vi "USB_test.vi"() -> ()   [LabVIEW 2024]
uses:
  <vilib>/Instr/_visa.llb/VISA Configure Serial Port (Instr).vi
panel:
  out "return count 2":u32
  in  "timeout (10sec)":u32=10000
  out "return count":u32
  out "error out":errorcluster
  out "read buffer":string
  in  "error in (no error)":errorcluster
  in  "VISA resource name":refnum<visa-resource-name>
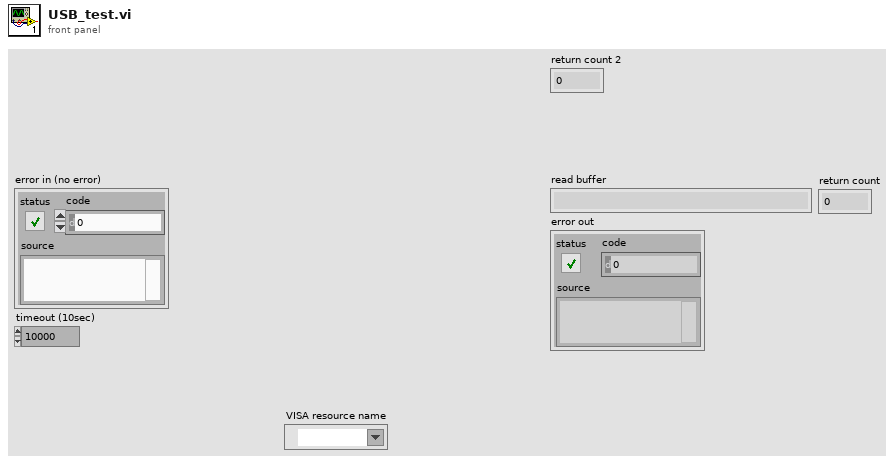
[diagram p1: front panel]
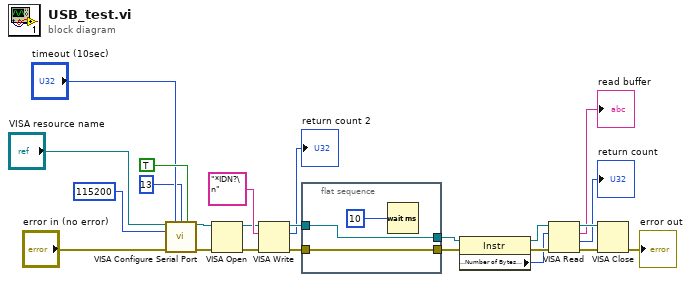
[diagram p0: block diagram]
diagram:
  n1 = call-poly "VISA Configure Serial Port"("VISA resource name"="VISA resource name", "timeout (10sec)"="timeout (10sec)", "termination char\n(0xA = '\\n' = LF)"=u8 13 ("termination char\n(0xA = '\\n' = LF)"), "Enable Termination\nChar (T)"=TRUE ("Enable Termination\nChar (T)"), "baud rate (9600)"=u32 115200, "error in (no error)"="error in (no error)") -> ("VISA resource name out"=w5:refnum<visa-resource-name>, "error out"=w6:errorcluster)  [unwired: 8 in]
  n2 = VISA Open(error in (no error)=w6, VISA resource name=w5) -> (VISA resource name=w4:refnum<visa-resource-name>, error out=w3:errorcluster)  [unwired: 3 in]
  n3 = VISA Write(VISA resource name=w4, write buffer="*IDN?\n", error in (no error)=w3) -> (VISA resource name out=w10:refnum<visa-resource-name>, return count=→"return count 2":u32, error out=w11:errorcluster)
  n4 = flat-sequence {
    tunnel: w10 -> [w27]
    tunnel: [w27] -> w16
    tunnel: w11 -> [w26]
    tunnel: [w26] -> w14
    frame #0 {
      n5 = Wait (ms)(milliseconds to wait=10) -> ()  [unwired: 1 out]
    }
  }
  n6 = property class="Instr"(reference=w16, error in=w14) -> (reference out=w15:refnum<visa-resource-name>, error out=w13:errorcluster, "Serial Settings:Number of Bytes at Serial Port"=w1:u32)
  n7 = VISA Read(VISA resource name=w15, byte count=w1, error in (no error)=w13) -> (VISA resource name out=w24:refnum<visa-resource-name>, read buffer=→"read buffer":string, return count=→"return count":u32, error out=w23:errorcluster)
  n8 = VISA Close(VISA resource name=w24, error in (no error)=w23) -> (error out=→"error out":errorcluster)
